vi "Eth Status Write Write Enable_com.vi"(7 "Status Reference":T1, 8 "error in (no error)":errorcluster, 9 "Write Enable":bool) -> (0 "error out":errorcluster)   [LabVIEW 2019, in "Eth Status.lvlib"]
uses:
  Eth Status.lvlib
  Ctl/Status.ctl
  MB_TCP2/MB_TCP_State.ctl
  MB_TCP2/MB_TCP.lvclass
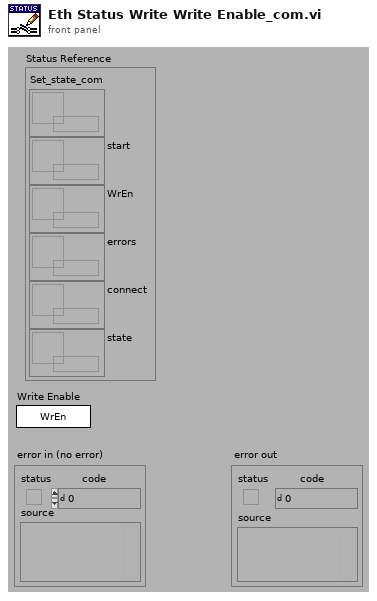
[diagram p1: front panel]
types:
  T1 = typedef "Eth Status.lvlib/Status.ctl" = cluster{"Set_state_com":refnum<data-value>, "start":refnum<data-value>, "WrEn":refnum<data-value>, "errors":refnum<data-value>, "connect":refnum<data-value>, "state":refnum<data-value>}
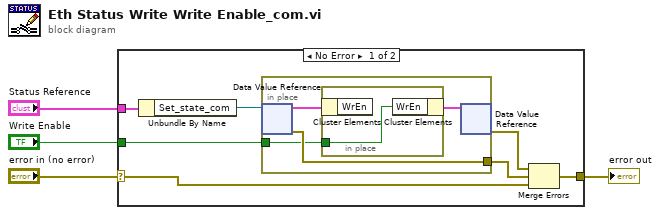
[diagram p0: block diagram]
diagram:
  n1 = case shown="No Error" "error in (no error)" {
    selector: "error in (no error)" -> [w9 w17]
    tunnel: [w10 w17] -> w4
    tunnel: "Status Reference" -> [w11 _]
    tunnel: "Write Enable" -> [w7 _]
    frame No Error {
      n2 = Unbundle By Name(w11) -> ("Set_state_com"=w8:refnum<data-value>)
      n3 = in-place {
        in-place-border: [w15] -> w5
        in-place-border: w7 -> [w13]
        n4 = in-place-dvr #1(w8) -> (w14:cluster{"Start":bool, "WrEn":bool, "Stop":bool}, w15:errorcluster)
        n5 = in-place {
          in-place-border: w13 -> [w16]
          n6 = in-place-cluster #2(w14) -> ()  [unwired: 1 out]
          n7 = in-place-cluster #2("WrEn"=w16) -> (w12:cluster{"Start":bool, "WrEn":bool, "Stop":bool})
        }
        n8 = in-place-dvr #1(w12) -> (w6:errorcluster)  [unwired: 1 out]
      }
      n9 = Merge Errors(w6, w5, w9) -> (w10:errorcluster)
    }
    frame Error {
    }
  }
  "error out" <- w4
